vi "Binary 읽기.vi"() -> ()   [LabVIEW 2014]
panel:
  out "데이터":dbl[](array[numeric])
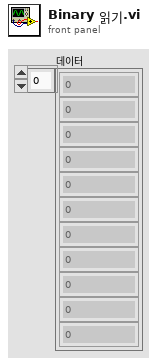
[diagram p1: front panel]
types:
  T1 = enum16{"open", "replace", "create", "open or create", "replace or create", "replace or create with confirmation"}
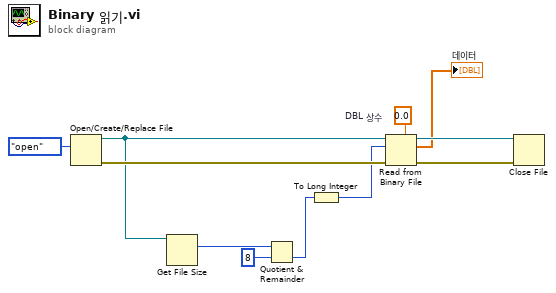
[diagram p0: block diagram]
diagram:
  w8 = 0.0  # DBL 상수
  n1 = Open/Create/Replace File(operation (0:open)=T1."open" ("동작(0:open)")) -> (refnum out=w6:refnum<file>, error out=w10:errorcluster)  [unwired: 5 in, 1 out]
  n2 = Get File Size(file=w6) -> (size (in bytes)=w5:i64)  [unwired: 1 in, 2 out]
  n3 = Quotient & Remainder(x=w5, y=i64 8) -> (floor(x/y)=w3:i64)  [unwired: 1 out]
  n4 = To Long Integer(number=w3) -> (32bit integer=w2:i32)
  n5 = Read from Binary File(5:w8, 8:w10, 10:w2, 11:w6) -> (0:w9:errorcluster, 2:→"데이터":dbl[], 3:w11:refnum<file>)  [unwired: 2 in, 1 out]
  n6 = Close File(refnum=w11, error in=w9) -> ()  [unwired: 2 out]
